vi "Test 1.vi"() -> ()   [LabVIEW 2015]
uses:
  source/xnode/Control-Refs.xnode
panel:
  out "Waveform Chart":dbl(graph)
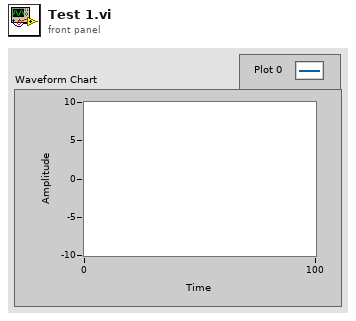
[diagram p1: front panel]
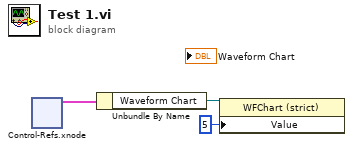
[diagram p0: block diagram]
diagram:
  n1 = xnode "Control-Refs.xnode"() -> ("Control Refs"=w1:cluster{"Waveform Chart":refnum<vi>})  [unwired: 1 in, 1 out]
  n2 = Unbundle By Name(w1) -> ("Waveform Chart"=w3:refnum<vi>)
  n3 = property class="WFChart (strict)"(reference=w3, "Value"=5) -> ()  [unwired: 1 in, 2 out]
